vi "test_OneSess_CallGetAllSession_ReturnsOneSession.vi"(8 "error in":errorcluster) -> (0 "error out":errorcluster, 2 "result":string, 3 "pass":bool)   [LabVIEW 2020, in "MeasurementServerTests.lvlib"]
uses:
  MeasurementServerTests.lvlib
  b3e5c3be-b7a7-4b6e-86ee-709eea9cb752.vi
  Runtime/MeasurementLink Session Management V1/Session Reservation/Session Reservation.lvclass
  Runtime/MeasurementLink Session Management V1/Session Reservation/Get Session Info - NSess .vi
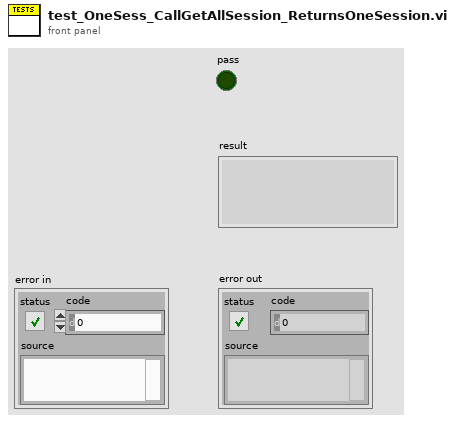
[diagram p1: front panel]
types:
  T1 = typedef "MeasurementLink Session Management V1.lvlib/Session Reservation.lvclass/Data.ctl" = cluster{"session and driver infos":T2[], "pin or relay names":string[], "connection map":refnum<class "Connection Map.lvclass">, "pin map context":T7, "reservation observer":refnum<class "IReservationObserver.lvclass">, "dvr valid":bool}
  T2 = typedef "MeasurementLink Session Management V1.lvlib/Session Reservation.lvclass/Session and Driver Info.ctl" = cluster{"session info":T3, "session":variant, "session factory":refnum<class "ISession Factory.lvclass">, "initialize and close session behavior":T6}
  T3 = typedef "MeasurementLink Session Management Client.lvlib/ni_measurementlink_sessionmanagement_v1_SessionInformation.ctl" = cluster{"session":T4, "resource_name":string, "channel_list":string, "instrument_type_id":string, "session_exists":bool, "channel_mappings":T5[]}
  T4 = typedef "MeasurementLink Session Management Client.lvlib/nidevice_grpc_Session.ctl" = cluster{"name":string}
  T5 = typedef "MeasurementLink Session Management Client.lvlib/ni_measurementlink_sessionmanagement_v1_ChannelMapping.ctl" = cluster{"pin_or_relay_name":string, "site":i32, "channel":string}
  T6 = typedef "MeasurementLink Instrument.lvlib/ISession Factory.lvclass/Initialize and Close Session Behavior.ctl" = enum16{"Initialize and Close", "Attach and Detach", "Initialize and Detach", "Attach and Close"}
  T7 = typedef "MeasurementLink Session Management Client.lvlib/ni_measurementlink_PinMapContext.ctl" = cluster{"pin_map_id":string, "sites":i32[]}
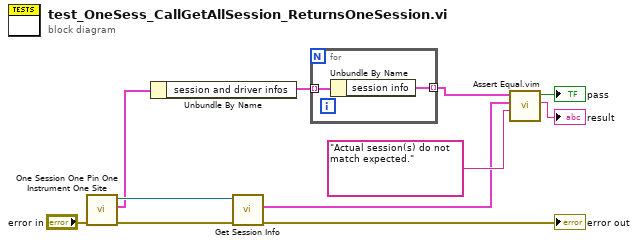
[diagram p0: block diagram]
diagram:
  n1 = call "One Session One Pin One Instrument One Site.vi"("error in"="error in") -> ("error out"=w3:errorcluster, "data out"=w1:T1, "session reservation out"=w2:refnum<class "Session Reservation.lvclass">)  [unwired: 8 in]
  n2 = Unbundle By Name(w1) -> ("session and driver infos"=w4:T2[])
  n3 = call-poly "Get Session Info.vi"("error in"=w3, "session reservation in"=w2) -> ("error out"=→"error out":errorcluster, "sessions info"=w6:T3[])  [unwired: 7 in, 1 out]
  n4 = for {
    tunnel: w4 -> [w13] mode=indexing
    tunnel: [w12] -> w5 mode=indexing
    n5 = Unbundle By Name(w13) -> ("session info"=w12:T3)
  }
  n6 = call "Assert Equal.vim"("failure message"="Actual session(s) do not match expected.", "actual value"=w6, "expected value"=w5) -> ("message"=→"result":string, "equal?"=→"pass":bool)  [unwired: 7 in]
